vi "HTTPMethod_Synchronous.vi"(0 "LabVIEWHTTPClient_NET in":refnum<class "HttpClient_NET.lvclass">, 2 "Method":T2, 3 "output file":path, 5 "URL":string, 7 "HttpContent":refnum<class "HttpContent.lvclass">, 9 "HttpRequestMessage":refnum<class "HttpRequestMessage.lvclass">, 11 "error in (no error)":errorcluster, 12 "Timeout_ms (10000)":i32=10000) -> (4 "LabVIEWHTTPClient_NET out":refnum<class "HttpClient_NET.lvclass">, 6 "Headers":T1, 8 "Response":string, 10 "StatusCode":i32(ring)=100 items=["Continue"=100, "SwitchingProtocols"=101, "OK"=200, "Created"=201, "Accepted"=202, "NonAuthoritativeInformation"=203, "NoContent"=204, "ResetContent"=205, "PartialContent"=206, "MultipleChoices, Ambiguous"=300, "MovedPermanently, Moved"=301, "Found, Redirect"=302, "SeeOther, RedirectMethod"=303, "NotModified"=304, "UseProxy"=305, "Unused"=306, "TemporaryRedirect, RedirectKeepVerb"=307, "BadRequest"=400, "Unauthorized"=401, "PaymentRequired"=402, "Forbidden"=403, "NotFound"=404, "MethodNotAllowed"=405, "NotAcceptable"=406, "ProxyAuthenticationRequired"=407, "RequestTimeout"=408, "Conflict"=409, "Gone"=410, "LengthRequired"=411, "PreconditionFailed"=412, "RequestEntityTooLarge"=413, "RequestUriTooLong"=414, "UnsupportedMediaType"=415, "RequestedRangeNotSatisfiable"=416, "ExpectationFailed"=417, "UpgradeRequired"=426, "InternalServerError"=500, "NotImplemented"=501, "BadGateway"=502, "ServiceUnavailable"=503, "GatewayTimeout"=504, "HttpVersionNotSupported"=505], 13 "ReasonPhrase":string, 14 "Timeout":bool, 15 "error out":errorcluster)   [LabVIEW 2018, in "HttpClient_NET.lvlib" / "HttpClient_NET.lvclass"]
doc: "<b> </b> <b> </b>\nHttpClient_NET\nJustin Young - Viviota\nCopyright (c) 2021\nLicense: BSD"
uses:
  HttpClient_NET.lvclass
  Types/method_enum.ctl
  HttpRequestMessage/HttpRequestMessage.lvclass
  HttpContent/HttpContent.lvclass
  Types/ResponseHeaders_Cluster.ctl
  HttpHeaders_response/HttpHeaders_Response.lvclass
  HttpHeaders_content/HttpHeaders_Content.lvclass
  HttpResponseMessage/HttpResponseMessage.lvclass
  HttpClient_NET.lvlib
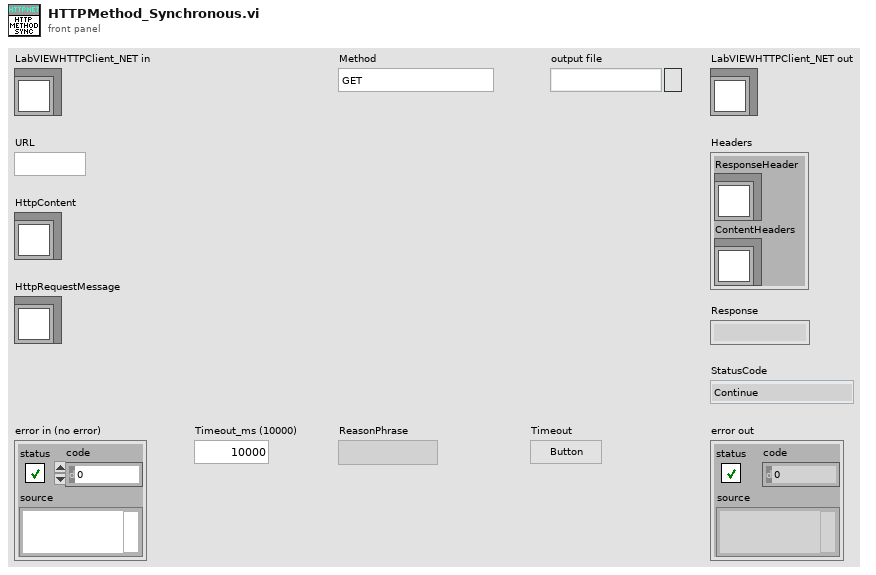
[diagram p1: front panel]
types:
  T1 = typedef "HttpClient_NET.lvlib/ResponseHeaders_Cluster.ctl" = cluster{"ResponseHeader":refnum<class "HttpHeaders_Response.lvclass">, "ContentHeaders":refnum<class "HttpHeaders_Content.lvclass">}
  T2 = typedef "HttpClient_NET.lvlib/method_enum.ctl" = enum16{"GET", "PUT", "POST", "DELETE", "HEAD", "TRACE", "SEND"}
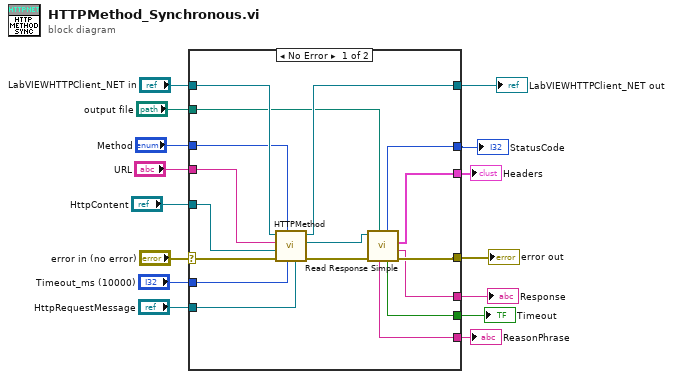
[diagram p0: block diagram]
diagram:
  n1 = case shown="No Error" "error in (no error)" {
    selector: "error in (no error)" -> [w32 w34]
    tunnel: [w23 w34] -> w14
    tunnel: [w25 w33] -> w12
    tunnel: "LabVIEWHTTPClient_NET in" -> [w29 w33]
    tunnel: "Method" -> [w28 _]
    tunnel: "Timeout_ms (10000)" -> [w31 _]
    tunnel: "URL" -> [w26 _]
    tunnel: "HttpContent" -> [w27 _]
    tunnel: "HttpRequestMessage" -> [w30 _]
    tunnel: "output file" -> [w21 _]
    tunnel: [w20 _] -> w5
    tunnel: [w19 _] -> w4
    tunnel: [w18 _] -> w2
    tunnel: [w17 _] -> w3
    tunnel: [w16 _] -> w1
    frame No Error {
      n2 = call "HTTPMethod.vi"("HttpRequestMessage"=w30, "Timeout_ms (10000)"=w31, "Method"=w28, "error in (no error)"=w32, "HttpContent"=w27, "URL"=w26, "LabVIEWHTTPClient_NET in"=w29) -> ("error out"=w24:errorcluster, "HttpResponseMessage out"=w22:refnum<class "HttpResponseMessage.lvclass">, "LabVIEWHTTPClient_NET out"=w25:refnum<class "HttpClient_NET.lvclass">)  [unwired: 2 in]
      n3 = call "Read Response Simple.vi"("output file"=w21, "error in (no error)"=w24, "HttpResponseMessage in"=w22) -> ("error out"=w23:errorcluster, "Response"=w19:string, "Headers"=w17:T1, "Timeout"=w20:bool, "StatusCode"=w18:i32, "ReasonPhrase"=w16:string)  [unwired: 3 in]
    }
    frame Error {
    }
  }
  "error out" <- w14
  "LabVIEWHTTPClient_NET out" <- w12
  "Timeout" <- w5
  "Response" <- w4
  "Headers" <- w3
  "StatusCode" <- w2
  "ReasonPhrase" <- w1
